vi "Convert to One-sided FFT（real）.vi"(1 "two-sided spectrum (real)":dbl[](array[numeric])) -> (0 "one-sided spectrum (real)":dbl[](array[numeric]))   [LabVIEW 2014]
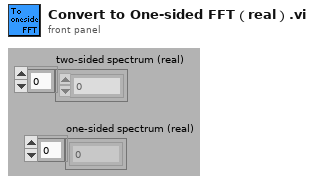
[diagram p1: front panel]
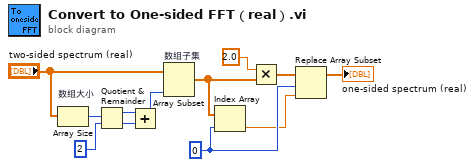
[diagram p0: block diagram]
diagram:
  w2 = 0 ("索引")
  n1 = Array Size "数组大小"(array="two-sided spectrum (real)") -> (size(s)=w10:i32)
  n2 = Quotient & Remainder(x=w10, y=2) -> (x-y*floor(x/y)=w8:i32, floor(x/y)=w12:i32)
  n3 = Add(x=w8, y=w12) -> (x+y=w7:i32)
  n4 = Array Subset "数组子集"(array="two-sided spectrum (real)", length=w7) -> (w5:dbl[])  [unwired: 1 in]
  n5 = Index Array(array=w5, index=w2) -> (element=w1:dbl)
  n6 = Multiply(x=2.0, y=w5) -> (x*y=w4:dbl[])
  n7 = Replace Array Subset(array=w4, new element=w1, index=w2) -> (→"one-sided spectrum (real)":dbl[])
